vi "UI.vi"(0 "reference in":refnum<class "GUI HIPRESS.lvclass">, 5 "error in (no error)":errorcluster) -> (14 "reference out":refnum<class "GUI HIPRESS.lvclass">, 19 "error out":errorcluster)   [LabVIEW 2019, in "GUI HIPRESS.lvclass"]
uses:
  GUI HIPRESS.lvclass
  GUI_class/GUI.lvclass
  D:/GIT H4000/H4000/src/GUI_class/GUI.lvclass
  d0ca9bf2-7cd9-4c29-a03d-de1c10393a74.vi
  MessageAMC_class/MessageAMC.lvclass
  c2a84178-5316-4673-968e-a9140ec84af1.vi
  7e6ae162-464c-44cf-a5e9-db9ce9dff507.vi
  143f14c2-2a31-4e71-909b-26881bbfe12c.vi
  modbus engine custom/MB_ENGINE_class/Settings.ctl
  modbus engine custom/MB_ENGINE_class/MB_ENGINE.lvclass
  TypeDef/Needle Valve State.ctl
  modbus engine custom/MB_ENGINE_class/Engine State.ctl
  modbus engine custom/MB_ENGINE_class/Engine Alarms.ctl
  TypeDef/Needle Valve Data.ctl
  modbus engine custom/MB_ENGINE_class/Limits Status.ctl
  TypeDef/Step_Name.ctl
  SV_Wrap/SharedVariableWrapper.lvclass
  MessageInterface_class/MessageInterface.lvclass
  b90cc415-26ee-4557-af2e-3b67e66185d6.vi
  TypeDef/AI Statistics Data.ctl
  TypeDef/AI_Data.ctl
  TypeDef/AI_Data_Array.ctl
  D:/GIT H4000/H4000/src/MessageInterface_class/MessageInterface.lvclass
panel:
  in  "Multicolumn Listbox":i32(listbox)=-1
  in  "set":bool
  in  "stop pmg":bool
  in  "start":bool
  in  "step 11":bool
  in  "step 10":bool
  in  "step 8":bool
  in  "step 7":bool
  in  "step 6":bool
  in  "step 5":bool
  in  "step 4":bool
  in  "step 3":bool
  in  "step 2":bool
  in  "step 1":bool
  out "Waveform Chart":T1(graph)
  in  "Setpoint":dbl caption="Уставка [бар]"
  out "Connect":bool
  in  "stop":bool
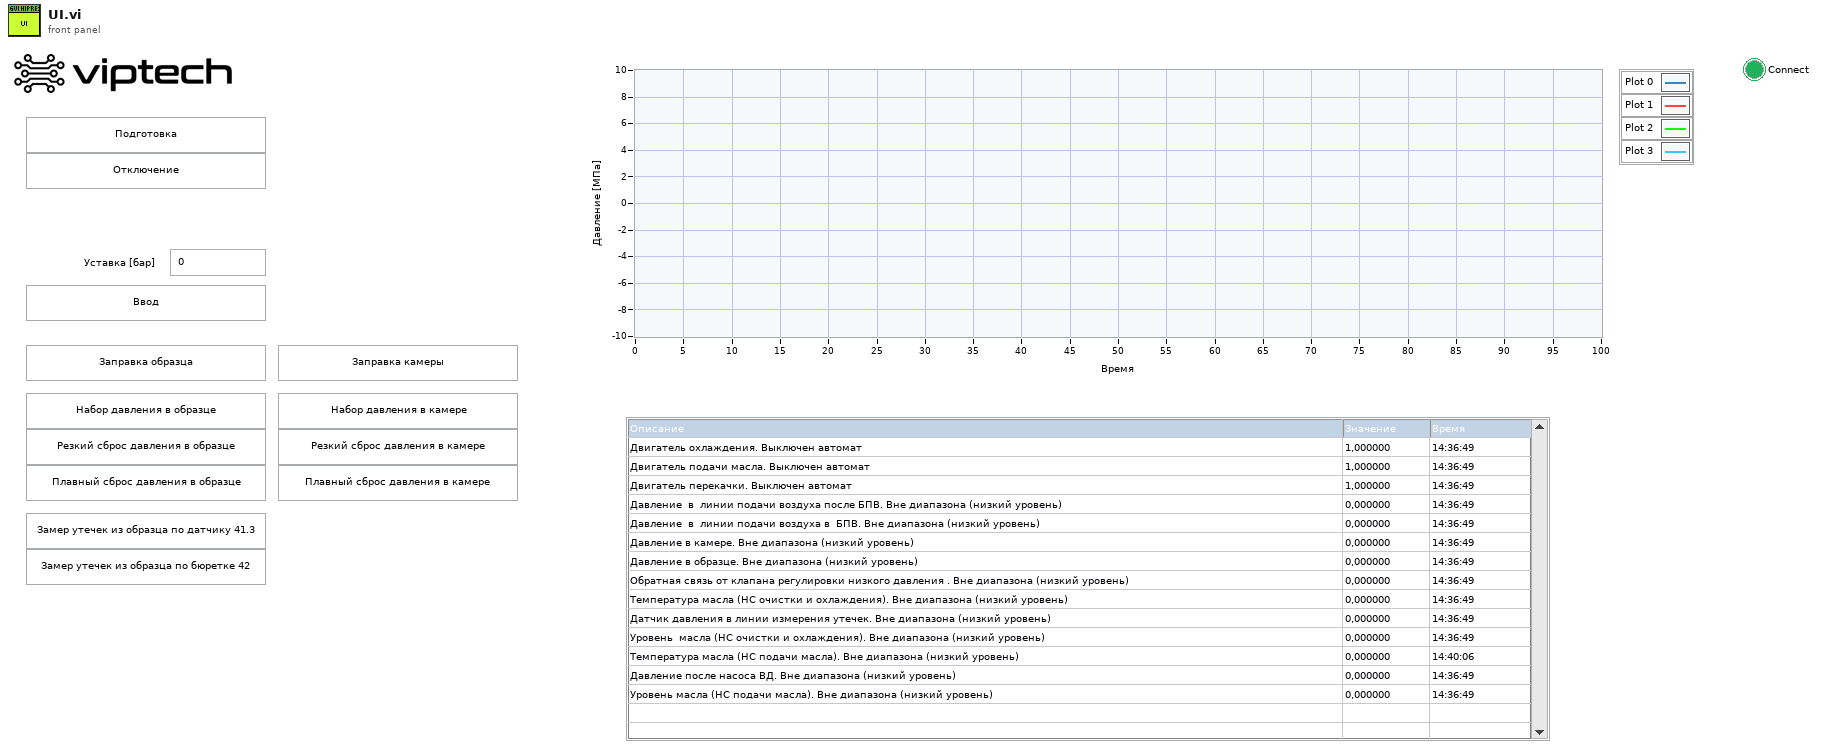
[diagram p1: front panel]
types:
  T1 = cluster{"Setpoint":dbl, "raw mean":dbl, "raw mean":dbl}
  T2 = typedef "Step_Name.ctl" = enum16{"NONE", "Filling DUT", "Filling Chamber", "Pressure Up DUT", "Abrupt Pressure Release DUT", "Smooth Pressure Release DUT", "Pressure Up Chamber", "Abrupt Pressure Release Chamber", "Smooth Pressure Release Chamber", "Measuring leakage sensor 41.3", "Measuring leakage burette 42", "Low Pressure DUT", "Low Pressure Chamber", "Low Pressure HPP", "ALARM", "Open Air", "MicroStep DUT", "MicroStep CMBR", "Stop Pump", "Press Down by Valve DUT"}
  T3 = enum32{"Invalid", "Standard", "Closed", "Hidden", "Minimized", "Maximized"}
  T4 = enum32{"invalid app kind", "Development System", "Run Time System", "Student Edition", "Embedded LabVIEW", "Evaluation", "Custom"}
  T5 = typedef "SharedVariableWrapper.lvclass/Config.ctl" = cluster{"connection str":string, "timeout":dbl, "ip":string}
  T6 = cluster{"Core":cluster{"Current VI Reference":refnum<vi>, "Close Panel on Exit?":bool}, "amc":refnum<class "MessageAMC.lvclass">}
  T7 = cluster{"Current VI Reference":refnum<vi>, "Close Panel on Exit?":bool}
  T8 = typedef "Needle Valve Data.ctl" = cluster{"Engine State":T9, "StateValveModbus":T10, "Alarms":T11, "RAW":i32, "Angele":dbl, "Step":i32, "Encoder":i32, "Kinematic":T12, "Limits":T13, "EncoderMax":i32, "Counter Max Dont Update":i32, "EncoderMin":i32, "Counter Min Dont Update":i32, "Prepere Counter":i32, "STEP INIT":i32, "offset - Angel":dbl}
  T9 = typedef "MB_ENGINE.lvclass/Engine State.ctl" = u16
  T10 = typedef "Needle Valve State.ctl" = enum16{"STOPED", "CLOSED", "OPENED", "OPENING", "CLOSING", "FULL_CLOSE"}
  T11 = typedef "MB_ENGINE.lvclass/Engine Alarms.ctl" = cluster{"OL":bool, "TF":bool, "STL":bool, "OCP":bool, "CPUV":bool, "UVLO":bool, "SPI_ERROR":bool, "Fault":bool, "OL 2":bool, "TF 2":bool, "STL 2":bool, "OCP 2":bool, "CPUV 2":bool, "UVLO 2":bool, "reserved":bool, "InitDone":bool}
  T12 = typedef "MB_ENGINE.lvclass/Settings.ctl" = cluster{"ACC Steps Per Sec^2":u16, "DEC Steps Per Sec^2":u16, "Min Velosity Step Per Sec":u16, "Max Velosity Step Per Sec":u16, "MicroStep":u16}
  T13 = typedef "MB_ENGINE.lvclass/Limits Status.ctl" = cluster{"Fault 2 Switch":bool, "Fault 1 Switch":bool, "Center(Home)":bool, "Lower Limit":bool, "Upper Limit":bool}
  T14 = typedef "AI_Data_Array.ctl" = T15[]
  T15 = typedef "AI_Data.ctl" = cluster{"Stat Data":T16, "OutOfRangeMax":bool, "OutOfRangeMin":bool, "HIHI":bool, "HI":bool, "LO":bool, "LOLO":bool}
  T16 = typedef "AI Statistics Data.ctl" = cluster{"raw mean":dbl, "scl mean":dbl, "raw mean 1Hz":dbl, "scl mean 1Hz":dbl}
  T17 = cluster{"Setpoint":dbl, "scl mean 1Hz":dbl, "scl mean 1Hz":dbl}
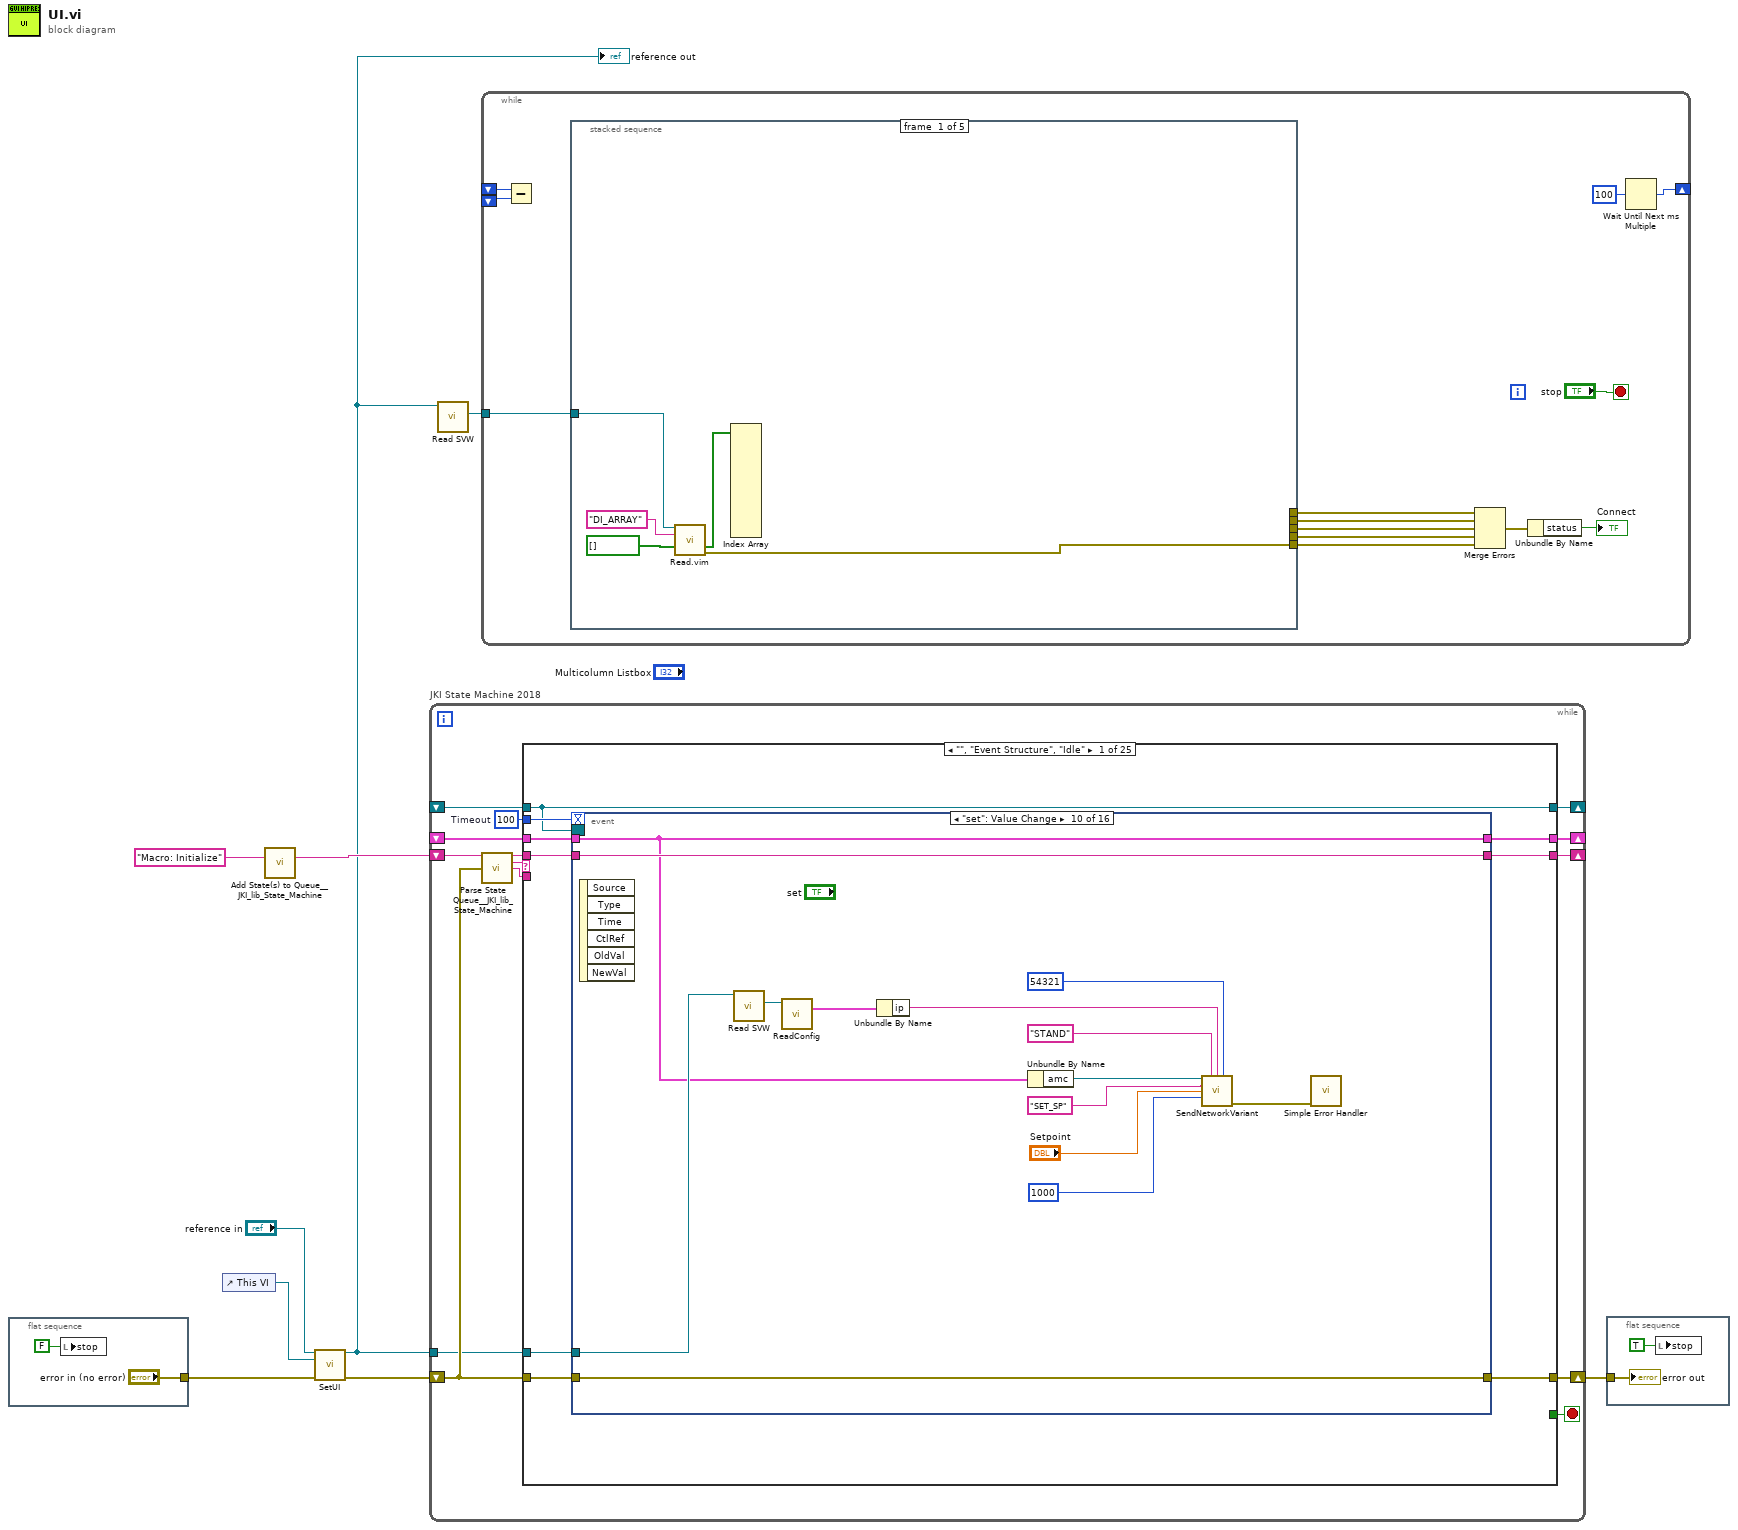
[diagram p0: block diagram]
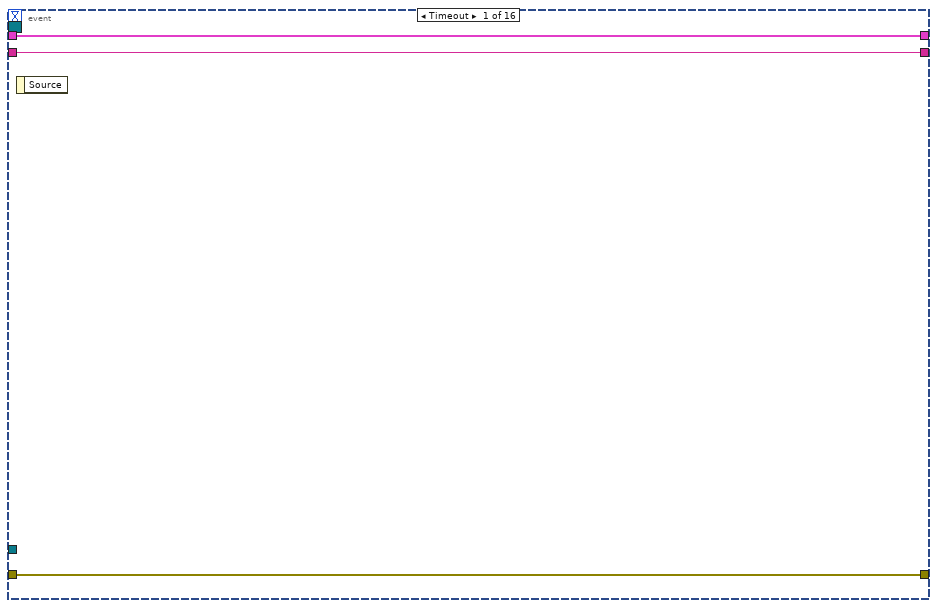
[diagram p2: hidden frame]
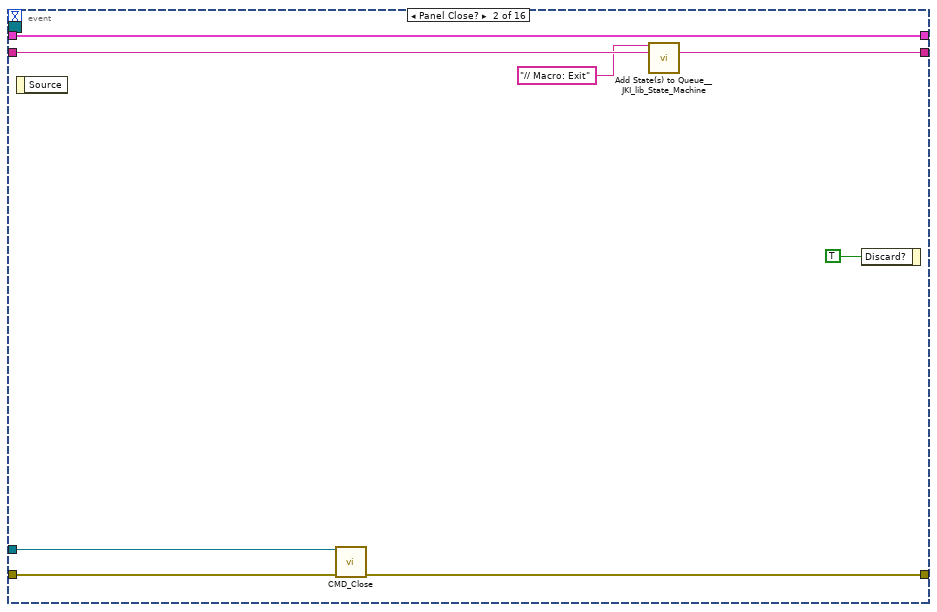
[diagram p3: hidden frame]
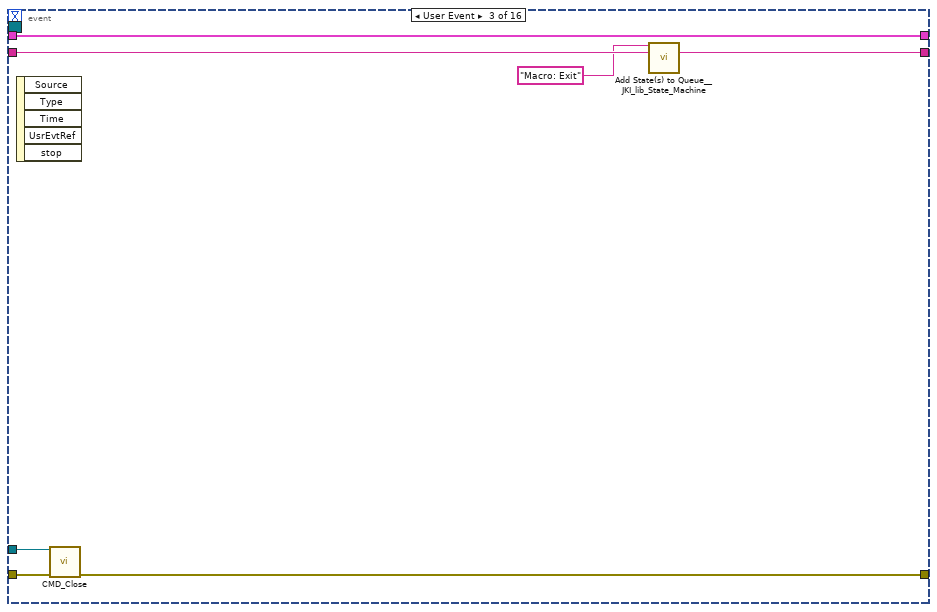
[diagram p4: hidden frame]
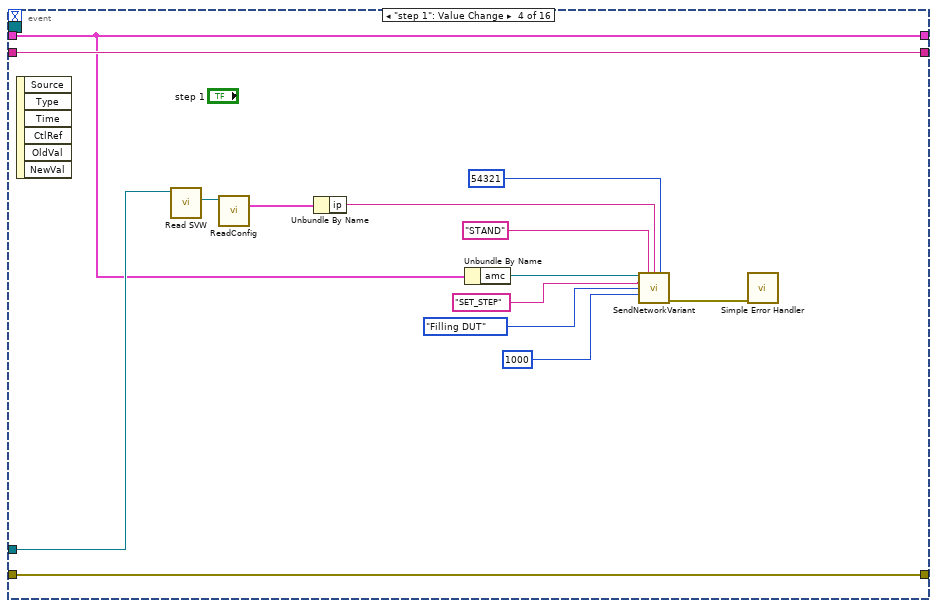
[diagram p5: hidden frame]
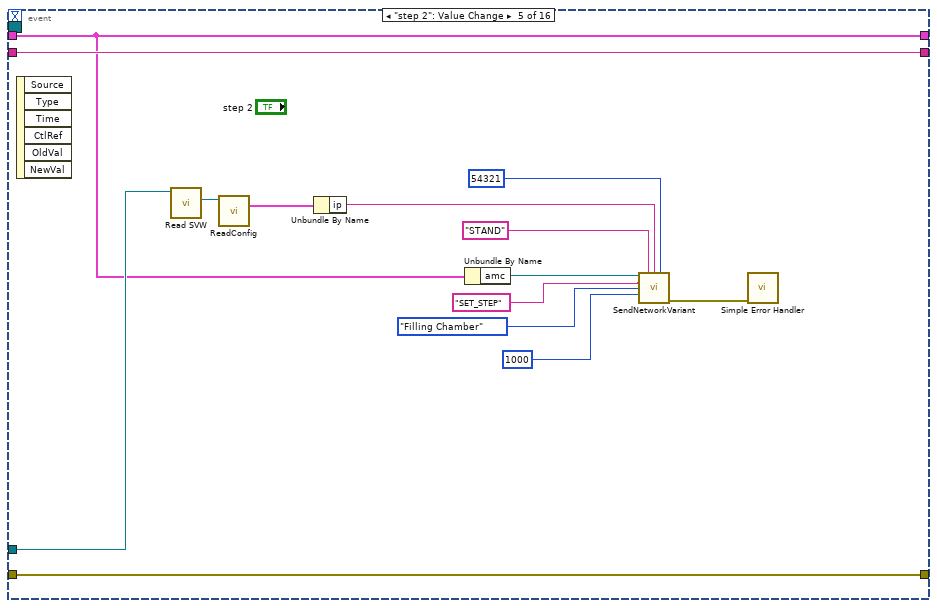
[diagram p6: hidden frame]
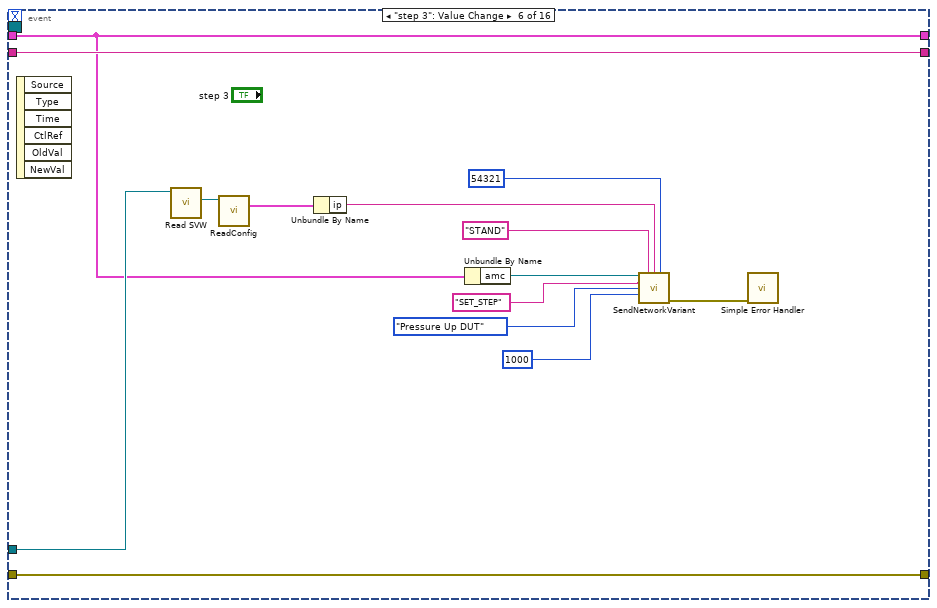
[diagram p7: hidden frame]
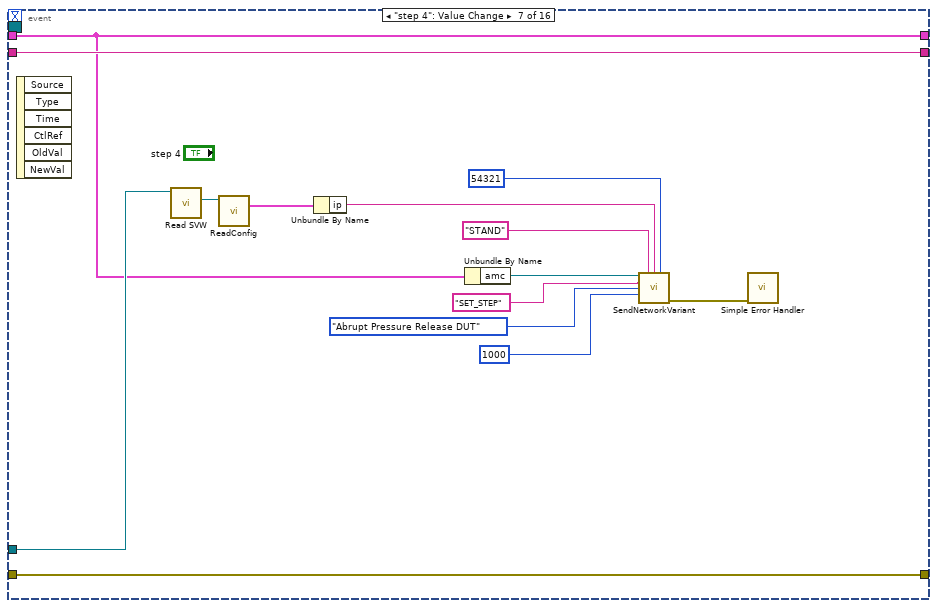
[diagram p8: hidden frame]
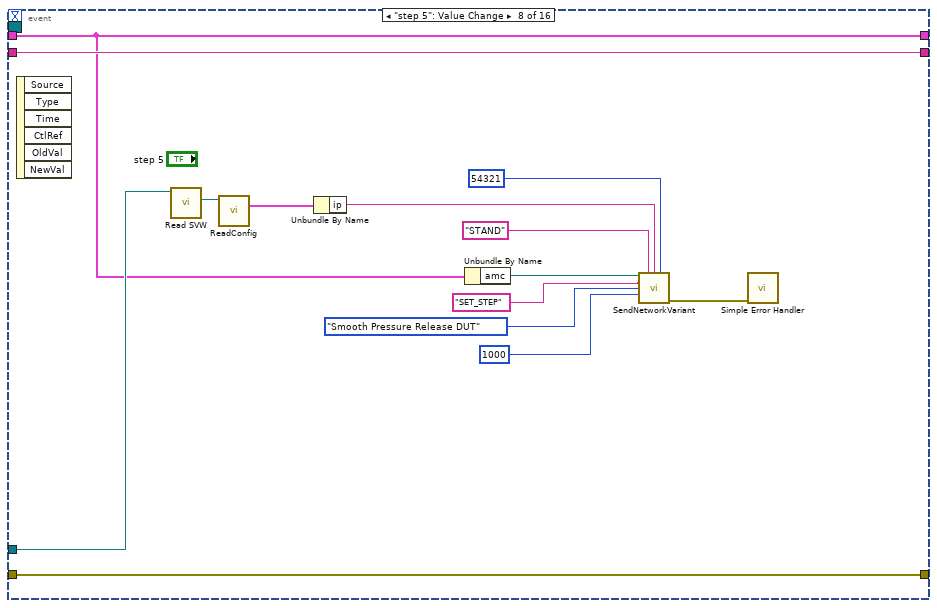
[diagram p9: hidden frame]
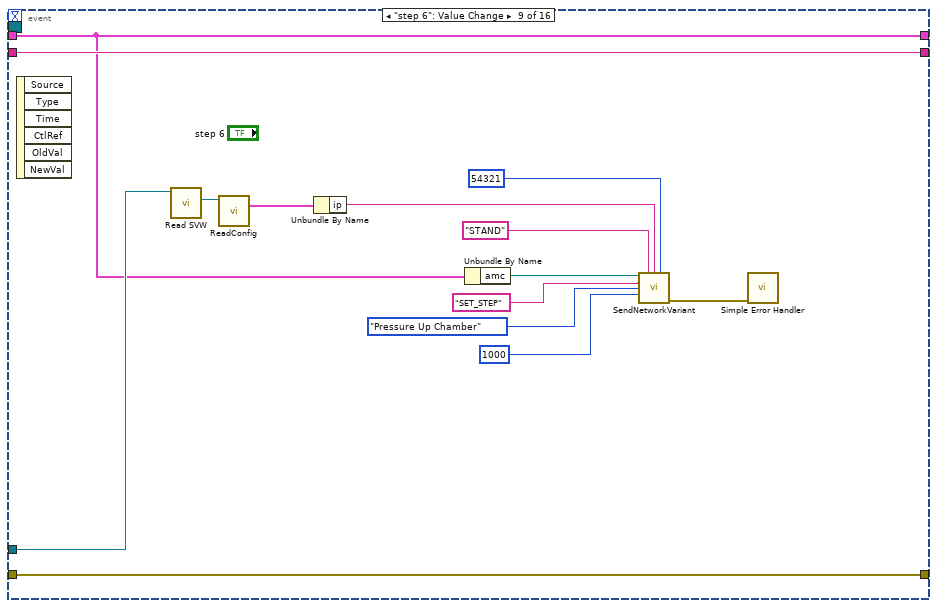
[diagram p10: hidden frame]
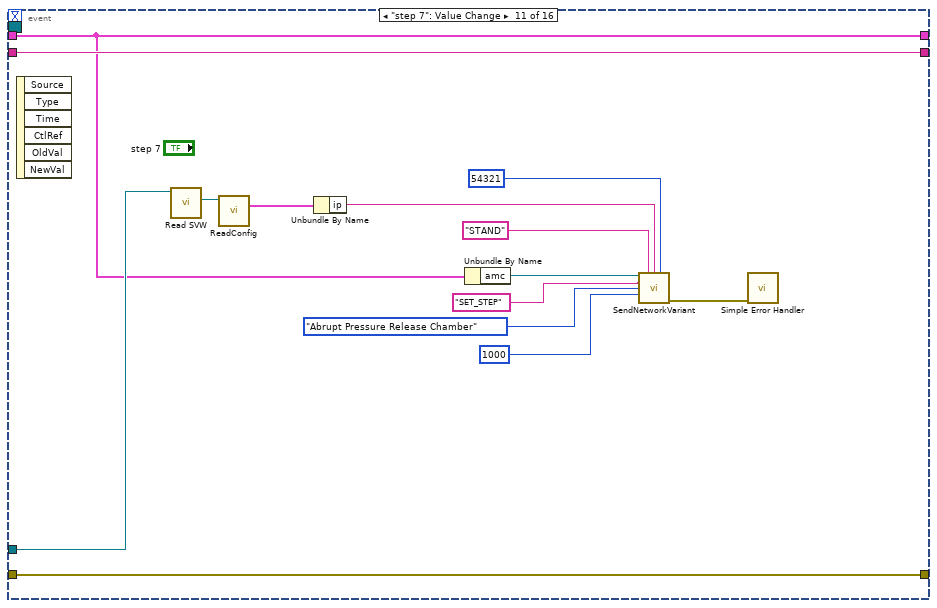
[diagram p11: hidden frame]
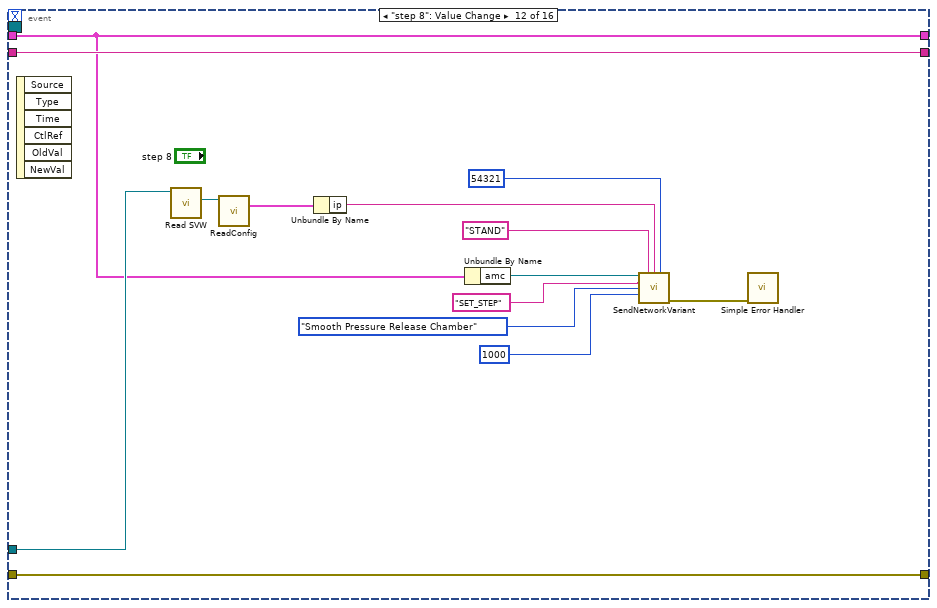
[diagram p12: hidden frame]
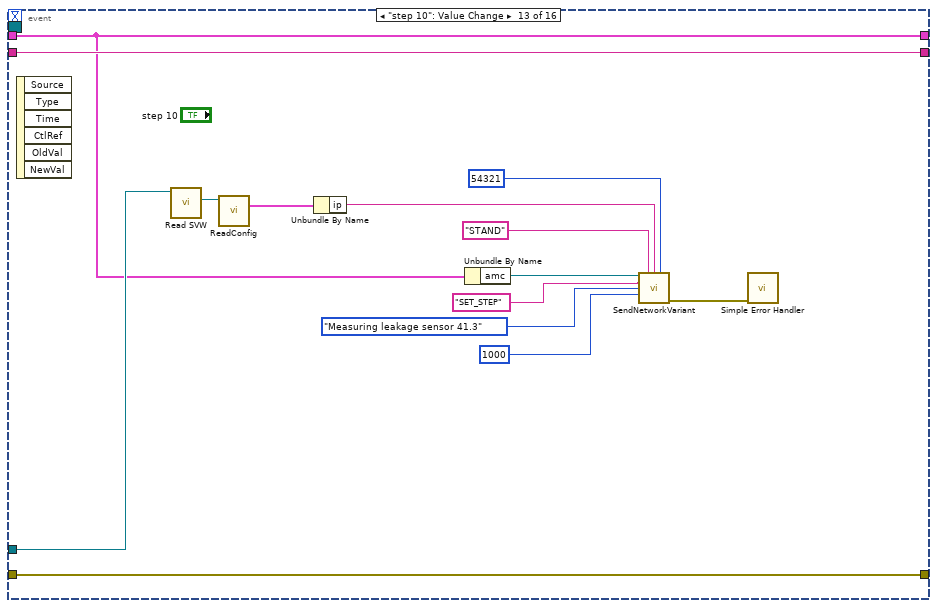
[diagram p13: hidden frame]
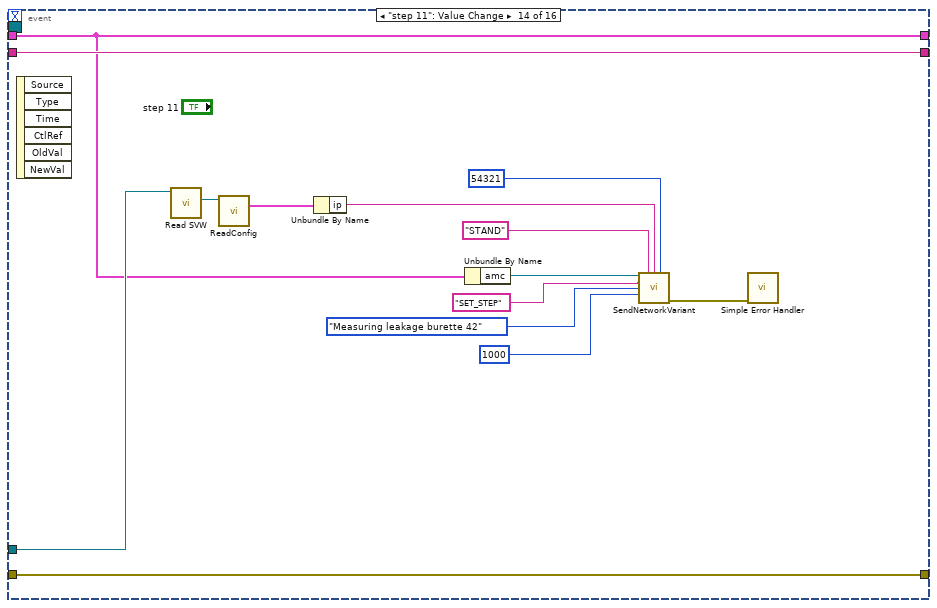
[diagram p14: hidden frame]
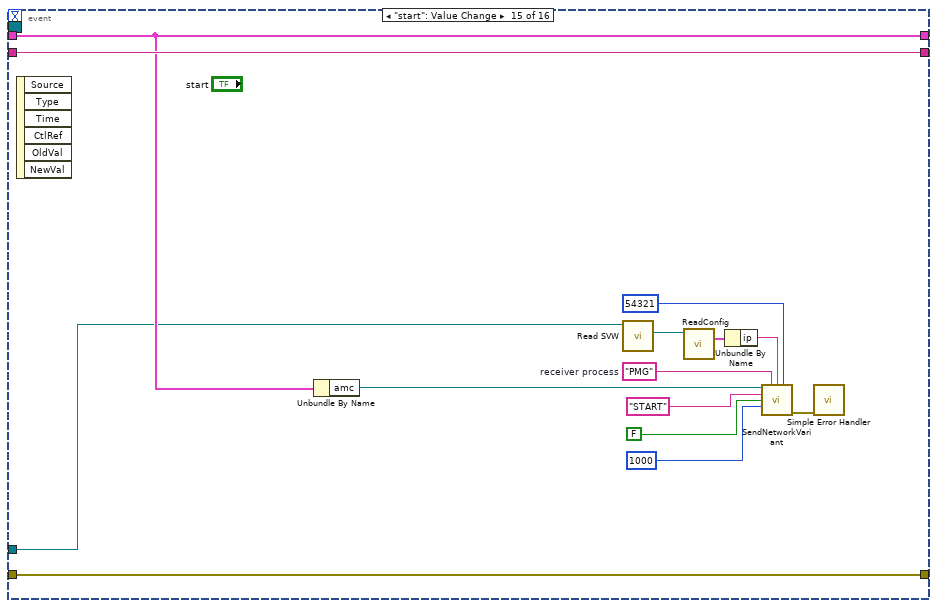
[diagram p15: hidden frame]
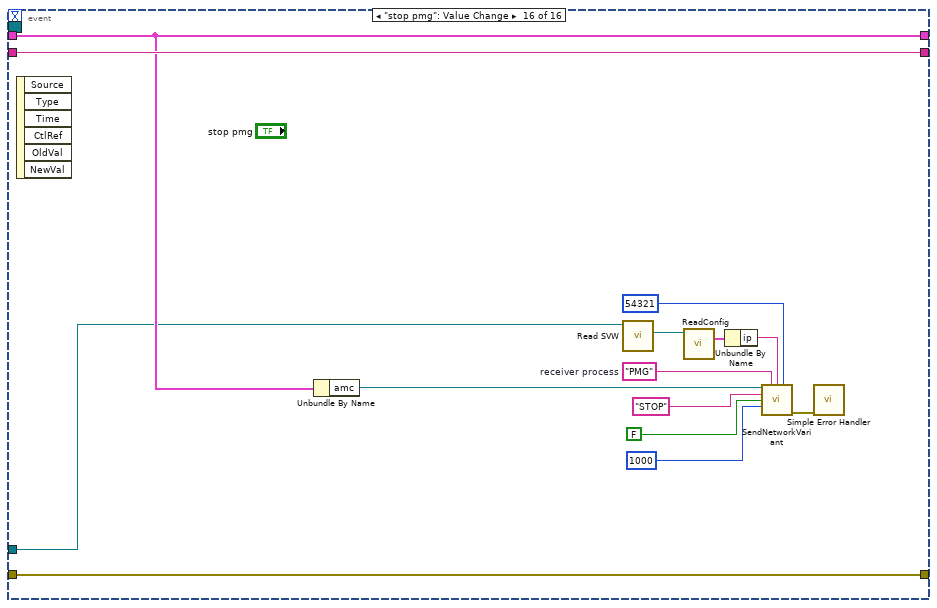
[diagram p16: hidden frame]
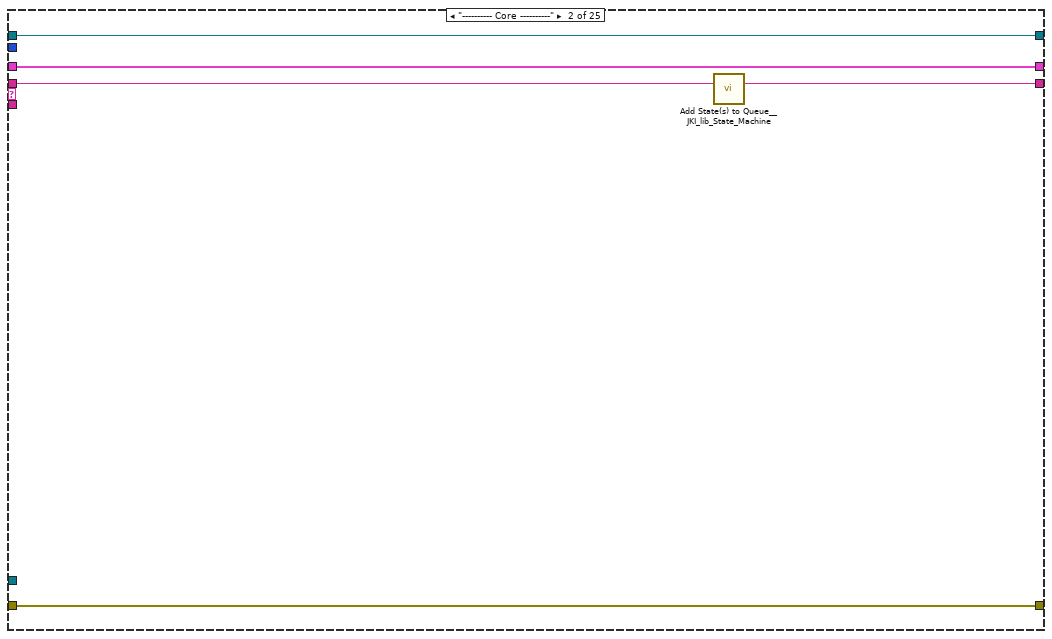
[diagram p17: hidden frame]
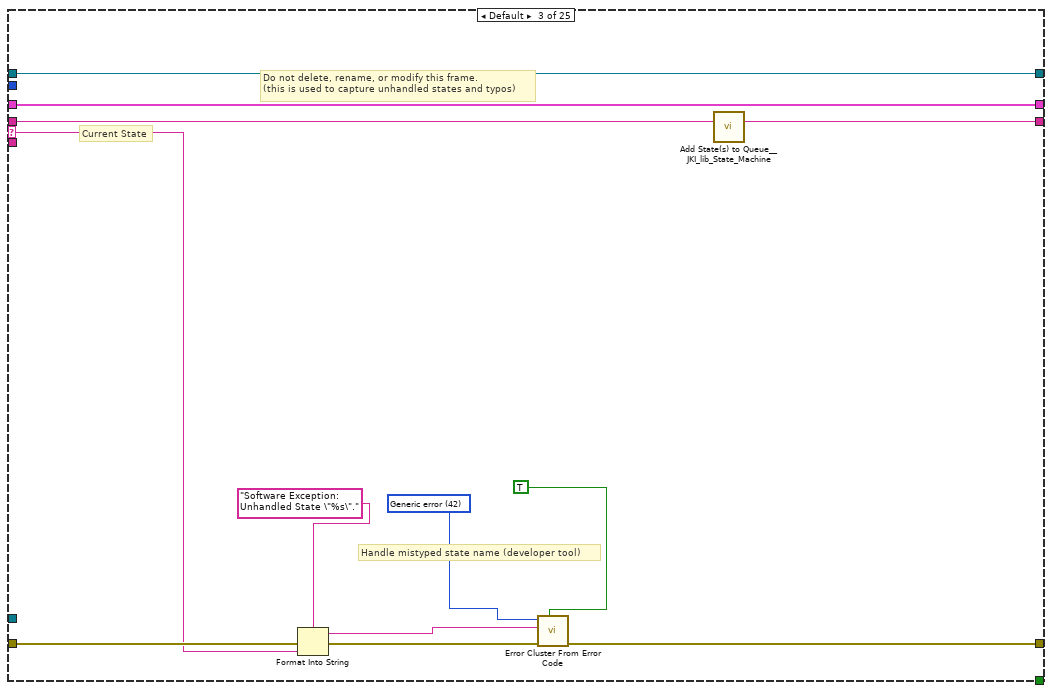
[diagram p18: hidden frame]
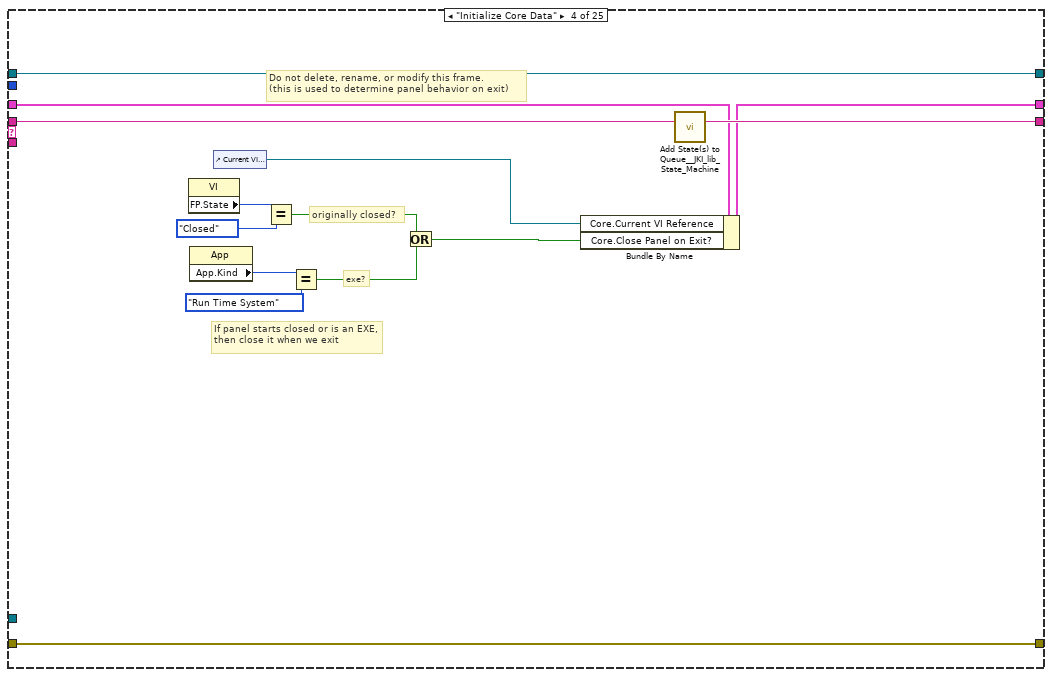
[diagram p19: hidden frame]
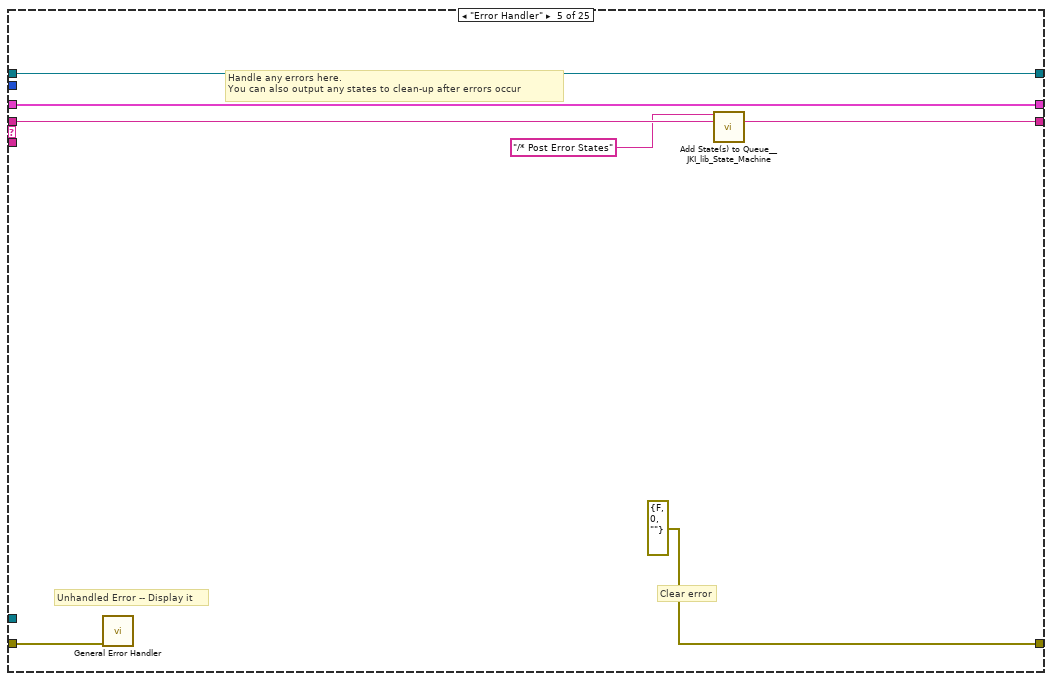
[diagram p20: hidden frame]
diagram:
  n1 = flat-sequence {
    tunnel: ["error in (no error)"] -> w6
    frame #0 {
      n2 = local write "stop"(FALSE ("stop")) -> ()
    }
  }
  n3 = control-ref of="This VI"() -> (w4:refnum<vi>)
  n4 = call <vilib>:"Add State(s) to Queue__JKI_lib_State_Machine.vi"("State(s) in (\"\")"="Macro: Initialize") -> ("States Out"=w9:string)  [unwired: 14 in]
  n5 = call "SetUI.vi"("reference in"="reference in", "UI VI"=w4, "error in (no error)"=w6) -> ("reference out"=w2:refnum<class "GUI HIPRESS.lvclass">, "error out"=w3:errorcluster)  [unwired: 11 in]
  "reference out" <- w2
  n6 = while "JKI State Machine 2018" {
    shift-right: [w18] -> _
    shift-left: _ -> [w17]
    shift-right: [w21] -> w7
    shift-left: w3 -> [w15]
    shift-right: [w20] -> _
    shift-left: w9 -> [w22]
    tunnel: w2 -> [w14]
    shift-right: [w13] -> _
    shift-left: _ -> [w12]
    stop <- w19 stop-if-true
    w16 = 100  # Timeout
    n7 = call <vilib>:"Parse State Queue__JKI_lib_State_Machine.vi"("State Queue"=w22, "Error In (no error)"=w15) -> ("Remaining States"=w24:string, "Current State"=w25:string, "Arguments"=w23:string)  [unwired: 11 in]
    n8 = case shown="\"\", \"Event Structure\", \"Idle\"" w25 {
      selector: w25 -> [_ _ w241 _ _ _ _ _ _ _ _ _ _ _ _ _ _ _ _ _ _ _ _ _ _]
      tunnel: w24 -> [w34 w239 w245 w265 w272 w280 w285 w294 w301 w306 w313 w319 w324 w328 w335 w347 w417 w423 w429 w441 w445 w446 w455 w459 w461]
      tunnel: w23 -> [_ _ _ _ _ _ _ _ _ _ _ _ _ _ w330 w341 _ _ _ _ _ _ _ _ _]
      tunnel: w17 -> [w32 w236 w243 w258 w269 w275 w282 _ w296 w303 w312 w317 w321 w327 w333 w343 w414 w420 w426 w438 w443 w448 w453 w456 w460]
      tunnel: [w31 w237 w247 w262 errorcluster {"status"=FALSE, "code"=0, "source"=""} ("error out") w278 w283 w287 w297 w304 w310 w314 w322 w326 w331 w344 w415 w421 w427 w439 w444 w449 w452 w457 w463] -> w21
      tunnel: w15 -> [w30 w237 w246 w262 w268 w278 w283 w288 w298 w304 w309 w315 w322 w326 w332 w345 w415 w421 w427 w439 w444 w449 w452 w457 w463]
      tunnel: [w33 w238 w244 w264 w271 w279 w284 w294 w300 w305 w313 w318 w323 w328 w334 w346 w416 w422 w428 w440 w445 w447 w455 w459 w461] -> w20
      tunnel: [_ _ _ _ _ TRUE _ _ _ _ _ _ _ _ _ _ _ _ _ _ _ _ _ _ _] -> w19
      tunnel: [w29 w236 w243 w263 w269 w275 w282 w293 w296 w303 w312 w317 w321 w327 w333 w343 w414 w420 w426 w438 w443 w448 w453 w456 w460] -> w18
      tunnel: w16 -> [w28 _ _ _ _ _ _ _ _ _ _ _ _ _ _ _ _ _ _ _ _ _ _ _ _]
      tunnel: w14 -> [w27 _ _ _ _ _ _ _ _ _ w308 _ _ _ _ _ _ _ _ _ _ w450 _ _ _]
      tunnel: [w26 w235 w240 w252 w266 w276 w281 w291 w295 w302 w311 w316 w320 w325 w329 w340 w413 w418 w424 w431 w442 w451 w454 w458 w462] -> w13
      tunnel: w12 -> [w26 w235 w240 w252 w266 w276 w281 w291 w295 w302 _ w316 w320 w325 w329 w340 w413 w418 w424 w431 w442 w451 w454 w458 w462]
      frame "", "Event Structure", "Idle" {
        n9 = event shown="[9] \"set\": Value Change" {
          selector: w26 -> [_ _ _ _ _ _ _ _ _ _ _ _ _ _ _ _]
          dyn-events: _ -> [_ _ _ _ _ _ _ _ _ _ _ _ _ _ _ _]
          timeout: w28 -> [_ _ _ _ _ _ _ _ _ _ _ _ _ _ _ _]
          tunnel: w34 -> [w37 w45 w52 w66 w80 w94 w108 w122 w136 w150 w164 w178 w192 w206 w220 w234]
          tunnel: [w37 w44 w51 w66 w80 w94 w108 w122 w136 w150 w164 w178 w192 w206 w220 w234] -> w33
          tunnel: w32 -> [w35 w43 w50 w60 w74 w88 w102 w116 w130 w144 w158 w172 w186 w200 w208 w222]
          tunnel: [w36 w38 w46 w65 w79 w93 w107 w121 w135 w149 w163 w177 w191 w205 w219 w233] -> w31
          tunnel: w30 -> [w36 w39 w47 w65 w79 w93 w107 w121 w135 w149 w163 w177 w191 w205 w219 w233]
          tunnel: [w35 w43 w50 w60 w74 w88 w102 w116 w130 w144 w158 w172 w186 w200 w208 w222] -> w29
          tunnel: w27 -> [_ w40 w48 w61 w75 w89 w103 w117 w131 w145 w159 w173 w187 w201 w207 w221]
          event Timeout {
            n10 = event-data() -> ()  [unwired: 1 in, 1 out]
          }
          event Panel Close? {
            n11 = event-data() -> ()  [unwired: 1 in, 1 out]
            n12 = call "CMD_Close.vi"("reference in"=w40, "error in (no error)"=w39) -> ("error out"=w38:errorcluster)  [unwired: 12 in, 1 out]
            n13 = call <vilib>:"Add State(s) to Queue__JKI_lib_State_Machine.vi"("State(s) in Front (\"\")"="// Macro: Exit", "State(s) in (\"\")"=w45) -> ("States Out"=w44:string)  [unwired: 13 in]
            n14 = event-data("Discard?"=TRUE) -> ()  [unwired: 1 in, 1 out]
          }
          event User Event {
            n15 = event-data() -> ()  [unwired: 1 in, 5 out]
            n16 = call "CMD_Close.vi"("reference in"=w48, "error in (no error)"=w47) -> ("error out"=w46:errorcluster)  [unwired: 12 in, 1 out]
            n17 = call <vilib>:"Add State(s) to Queue__JKI_lib_State_Machine.vi"("State(s) in Front (\"\")"="Macro: Exit", "State(s) in (\"\")"=w52) -> ("States Out"=w51:string)  [unwired: 13 in]
          }
          event "step 1": Value Change {
            n18 = event-data() -> ()  [unwired: 1 in, 6 out]
            n19 = call "Read SVW.vi"("GUI in"=w61) -> ("SharedVariableWrapper.lvclass"=w64:refnum<class "SharedVariableWrapper.lvclass">)  [unwired: 10 in]
            n20 = call "ReadConfig.vi"("SharedVariableWrapper in"=w64) -> ("config"=w63:T5)  [unwired: 12 in, 2 out]
            n21 = Unbundle By Name(w63) -> ("ip"=w62:string)
            n22 = Unbundle By Name(w60) -> ("amc"=w59:refnum<class "MessageAMC.lvclass">)
            n23 = call "SendNetworkVariant.vi"("reference in"=w59, "receiver process"="STAND", "receiver host"=w62, "receiver port (0)"=u16 54321, "name"="SET_STEP", "data"=Step_Name."Filling DUT" ("stepName"), "timeout (25000 ms)"=1000) -> ("error out"=w56:errorcluster)  [unwired: 6 in, 2 out]
            n24 = call <vilib>:"Simple Error Handler.vi"("error in (no error)"=w56) -> ()  [unwired: 4 in, 5 out]
          }
          event "step 2": Value Change {
            n25 = event-data() -> ()  [unwired: 1 in, 6 out]
            n26 = call "Read SVW.vi"("GUI in"=w75) -> ("SharedVariableWrapper.lvclass"=w78:refnum<class "SharedVariableWrapper.lvclass">)  [unwired: 10 in]
            n27 = call "ReadConfig.vi"("SharedVariableWrapper in"=w78) -> ("config"=w77:T5)  [unwired: 12 in, 2 out]
            n28 = Unbundle By Name(w77) -> ("ip"=w76:string)
            n29 = Unbundle By Name(w74) -> ("amc"=w73:refnum<class "MessageAMC.lvclass">)
            n30 = call "SendNetworkVariant.vi"("reference in"=w73, "receiver process"="STAND", "receiver host"=w76, "receiver port (0)"=u16 54321, "name"="SET_STEP", "data"=Step_Name."Filling Chamber" ("stepName"), "timeout (25000 ms)"=1000) -> ("error out"=w70:errorcluster)  [unwired: 6 in, 2 out]
            n31 = call <vilib>:"Simple Error Handler.vi"("error in (no error)"=w70) -> ()  [unwired: 4 in, 5 out]
          }
          event "step 3": Value Change {
            n32 = event-data() -> ()  [unwired: 1 in, 6 out]
            n33 = call "Read SVW.vi"("GUI in"=w89) -> ("SharedVariableWrapper.lvclass"=w92:refnum<class "SharedVariableWrapper.lvclass">)  [unwired: 10 in]
            n34 = call "ReadConfig.vi"("SharedVariableWrapper in"=w92) -> ("config"=w91:T5)  [unwired: 12 in, 2 out]
            n35 = Unbundle By Name(w91) -> ("ip"=w90:string)
            n36 = Unbundle By Name(w88) -> ("amc"=w87:refnum<class "MessageAMC.lvclass">)
            n37 = call "SendNetworkVariant.vi"("reference in"=w87, "receiver process"="STAND", "receiver host"=w90, "receiver port (0)"=u16 54321, "name"="SET_STEP", "data"=Step_Name."Pressure Up DUT" ("stepName"), "timeout (25000 ms)"=1000) -> ("error out"=w84:errorcluster)  [unwired: 6 in, 2 out]
            n38 = call <vilib>:"Simple Error Handler.vi"("error in (no error)"=w84) -> ()  [unwired: 4 in, 5 out]
          }
          event "step 4": Value Change {
            n39 = event-data() -> ()  [unwired: 1 in, 6 out]
            n40 = call "Read SVW.vi"("GUI in"=w103) -> ("SharedVariableWrapper.lvclass"=w106:refnum<class "SharedVariableWrapper.lvclass">)  [unwired: 10 in]
            n41 = call "ReadConfig.vi"("SharedVariableWrapper in"=w106) -> ("config"=w105:T5)  [unwired: 12 in, 2 out]
            n42 = Unbundle By Name(w105) -> ("ip"=w104:string)
            n43 = Unbundle By Name(w102) -> ("amc"=w101:refnum<class "MessageAMC.lvclass">)
            n44 = call "SendNetworkVariant.vi"("reference in"=w101, "receiver process"="STAND", "receiver host"=w104, "receiver port (0)"=u16 54321, "name"="SET_STEP", "data"=Step_Name."Abrupt Pressure Release DUT" ("stepName"), "timeout (25000 ms)"=1000) -> ("error out"=w98:errorcluster)  [unwired: 6 in, 2 out]
            n45 = call <vilib>:"Simple Error Handler.vi"("error in (no error)"=w98) -> ()  [unwired: 4 in, 5 out]
          }
          event "step 5": Value Change {
            n46 = event-data() -> ()  [unwired: 1 in, 6 out]
            n47 = call "Read SVW.vi"("GUI in"=w117) -> ("SharedVariableWrapper.lvclass"=w120:refnum<class "SharedVariableWrapper.lvclass">)  [unwired: 10 in]
            n48 = call "ReadConfig.vi"("SharedVariableWrapper in"=w120) -> ("config"=w119:T5)  [unwired: 12 in, 2 out]
            n49 = Unbundle By Name(w119) -> ("ip"=w118:string)
            n50 = Unbundle By Name(w116) -> ("amc"=w115:refnum<class "MessageAMC.lvclass">)
            n51 = call "SendNetworkVariant.vi"("reference in"=w115, "receiver process"="STAND", "receiver host"=w118, "receiver port (0)"=u16 54321, "name"="SET_STEP", "data"=Step_Name."Smooth Pressure Release DUT" ("stepName"), "timeout (25000 ms)"=1000) -> ("error out"=w112:errorcluster)  [unwired: 6 in, 2 out]
            n52 = call <vilib>:"Simple Error Handler.vi"("error in (no error)"=w112) -> ()  [unwired: 4 in, 5 out]
          }
          event "step 6": Value Change {
            n53 = event-data() -> ()  [unwired: 1 in, 6 out]
            n54 = call "Read SVW.vi"("GUI in"=w131) -> ("SharedVariableWrapper.lvclass"=w134:refnum<class "SharedVariableWrapper.lvclass">)  [unwired: 10 in]
            n55 = call "ReadConfig.vi"("SharedVariableWrapper in"=w134) -> ("config"=w133:T5)  [unwired: 12 in, 2 out]
            n56 = Unbundle By Name(w133) -> ("ip"=w132:string)
            n57 = Unbundle By Name(w130) -> ("amc"=w129:refnum<class "MessageAMC.lvclass">)
            n58 = call "SendNetworkVariant.vi"("reference in"=w129, "receiver process"="STAND", "receiver host"=w132, "receiver port (0)"=u16 54321, "name"="SET_STEP", "data"=Step_Name."Pressure Up Chamber" ("stepName"), "timeout (25000 ms)"=1000) -> ("error out"=w126:errorcluster)  [unwired: 6 in, 2 out]
            n59 = call <vilib>:"Simple Error Handler.vi"("error in (no error)"=w126) -> ()  [unwired: 4 in, 5 out]
          }
          event "set": Value Change {
            n60 = event-data() -> ()  [unwired: 1 in, 6 out]
            n61 = call "Read SVW.vi"("GUI in"=w145) -> ("SharedVariableWrapper.lvclass"=w148:refnum<class "SharedVariableWrapper.lvclass">)  [unwired: 10 in]
            n62 = call "ReadConfig.vi"("SharedVariableWrapper in"=w148) -> ("config"=w147:T5)  [unwired: 12 in, 2 out]
            n63 = Unbundle By Name(w147) -> ("ip"=w146:string)
            n64 = Unbundle By Name(w144) -> ("amc"=w143:refnum<class "MessageAMC.lvclass">)
            n65 = call "SendNetworkVariant.vi"("reference in"=w143, "receiver process"="STAND", "receiver host"=w146, "receiver port (0)"=u16 54321, "name"="SET_SP", "data"="Setpoint", "timeout (25000 ms)"=1000) -> ("error out"=w140:errorcluster)  [unwired: 6 in, 2 out]
            n66 = call <vilib>:"Simple Error Handler.vi"("error in (no error)"=w140) -> ()  [unwired: 4 in, 5 out]
          }
          event "step 7": Value Change {
            n67 = event-data() -> ()  [unwired: 1 in, 6 out]
            n68 = call "Read SVW.vi"("GUI in"=w159) -> ("SharedVariableWrapper.lvclass"=w162:refnum<class "SharedVariableWrapper.lvclass">)  [unwired: 10 in]
            n69 = call "ReadConfig.vi"("SharedVariableWrapper in"=w162) -> ("config"=w161:T5)  [unwired: 12 in, 2 out]
            n70 = Unbundle By Name(w161) -> ("ip"=w160:string)
            n71 = Unbundle By Name(w158) -> ("amc"=w157:refnum<class "MessageAMC.lvclass">)
            n72 = call "SendNetworkVariant.vi"("reference in"=w157, "receiver process"="STAND", "receiver host"=w160, "receiver port (0)"=u16 54321, "name"="SET_STEP", "data"=Step_Name."Abrupt Pressure Release Chamber" ("stepName"), "timeout (25000 ms)"=1000) -> ("error out"=w154:errorcluster)  [unwired: 6 in, 2 out]
            n73 = call <vilib>:"Simple Error Handler.vi"("error in (no error)"=w154) -> ()  [unwired: 4 in, 5 out]
          }
          event "step 8": Value Change {
            n74 = event-data() -> ()  [unwired: 1 in, 6 out]
            n75 = call "Read SVW.vi"("GUI in"=w173) -> ("SharedVariableWrapper.lvclass"=w176:refnum<class "SharedVariableWrapper.lvclass">)  [unwired: 10 in]
            n76 = call "ReadConfig.vi"("SharedVariableWrapper in"=w176) -> ("config"=w175:T5)  [unwired: 12 in, 2 out]
            n77 = Unbundle By Name(w175) -> ("ip"=w174:string)
            n78 = Unbundle By Name(w172) -> ("amc"=w171:refnum<class "MessageAMC.lvclass">)
            n79 = call "SendNetworkVariant.vi"("reference in"=w171, "receiver process"="STAND", "receiver host"=w174, "receiver port (0)"=u16 54321, "name"="SET_STEP", "data"=Step_Name."Smooth Pressure Release Chamber" ("stepName"), "timeout (25000 ms)"=1000) -> ("error out"=w168:errorcluster)  [unwired: 6 in, 2 out]
            n80 = call <vilib>:"Simple Error Handler.vi"("error in (no error)"=w168) -> ()  [unwired: 4 in, 5 out]
          }
          event "step 10": Value Change {
            n81 = event-data() -> ()  [unwired: 1 in, 6 out]
            n82 = call "Read SVW.vi"("GUI in"=w187) -> ("SharedVariableWrapper.lvclass"=w190:refnum<class "SharedVariableWrapper.lvclass">)  [unwired: 10 in]
            n83 = call "ReadConfig.vi"("SharedVariableWrapper in"=w190) -> ("config"=w189:T5)  [unwired: 12 in, 2 out]
            n84 = Unbundle By Name(w189) -> ("ip"=w188:string)
            n85 = Unbundle By Name(w186) -> ("amc"=w185:refnum<class "MessageAMC.lvclass">)
            n86 = call "SendNetworkVariant.vi"("reference in"=w185, "receiver process"="STAND", "receiver host"=w188, "receiver port (0)"=u16 54321, "name"="SET_STEP", "data"=Step_Name."Measuring leakage sensor 41.3" ("stepName"), "timeout (25000 ms)"=1000) -> ("error out"=w182:errorcluster)  [unwired: 6 in, 2 out]
            n87 = call <vilib>:"Simple Error Handler.vi"("error in (no error)"=w182) -> ()  [unwired: 4 in, 5 out]
          }
          event "step 11": Value Change {
            n88 = event-data() -> ()  [unwired: 1 in, 6 out]
            n89 = call "Read SVW.vi"("GUI in"=w201) -> ("SharedVariableWrapper.lvclass"=w204:refnum<class "SharedVariableWrapper.lvclass">)  [unwired: 10 in]
            n90 = call "ReadConfig.vi"("SharedVariableWrapper in"=w204) -> ("config"=w203:T5)  [unwired: 12 in, 2 out]
            n91 = Unbundle By Name(w203) -> ("ip"=w202:string)
            n92 = Unbundle By Name(w200) -> ("amc"=w199:refnum<class "MessageAMC.lvclass">)
            n93 = call "SendNetworkVariant.vi"("reference in"=w199, "receiver process"="STAND", "receiver host"=w202, "receiver port (0)"=u16 54321, "name"="SET_STEP", "data"=Step_Name."Measuring leakage burette 42" ("stepName"), "timeout (25000 ms)"=1000) -> ("error out"=w196:errorcluster)  [unwired: 6 in, 2 out]
            n94 = call <vilib>:"Simple Error Handler.vi"("error in (no error)"=w196) -> ()  [unwired: 4 in, 5 out]
          }
          event "start": Value Change {
            w209 = "PMG"  # receiver process
            n95 = event-data() -> ()  [unwired: 1 in, 6 out]
            n96 = Unbundle By Name(w208) -> ("amc"=w213:refnum<class "MessageAMC.lvclass">)
            n97 = call "Read SVW.vi"("GUI in"=w207) -> ("SharedVariableWrapper.lvclass"=w215:refnum<class "SharedVariableWrapper.lvclass">)  [unwired: 10 in]
            n98 = call "ReadConfig.vi"("SharedVariableWrapper in"=w215) -> ("config"=w214:T5)  [unwired: 12 in, 2 out]
            n99 = Unbundle By Name(w214) -> ("ip"=w212:string)
            n100 = call "SendNetworkVariant.vi"("reference in"=w213, "receiver process"=w209, "receiver host"=w212, "receiver port (0)"=u16 54321, "name"="START", "data"=FALSE, "timeout (25000 ms)"=1000) -> ("error out"=w210:errorcluster)  [unwired: 6 in, 2 out]
            n101 = call <vilib>:"Simple Error Handler.vi"("error in (no error)"=w210) -> ()  [unwired: 4 in, 5 out]
          }
          event "stop pmg": Value Change {
            w223 = "PMG"  # receiver process
            n102 = event-data() -> ()  [unwired: 1 in, 6 out]
            n103 = Unbundle By Name(w222) -> ("amc"=w227:refnum<class "MessageAMC.lvclass">)
            n104 = call "Read SVW.vi"("GUI in"=w221) -> ("SharedVariableWrapper.lvclass"=w229:refnum<class "SharedVariableWrapper.lvclass">)  [unwired: 10 in]
            n105 = call "ReadConfig.vi"("SharedVariableWrapper in"=w229) -> ("config"=w228:T5)  [unwired: 12 in, 2 out]
            n106 = Unbundle By Name(w228) -> ("ip"=w226:string)
            n107 = call "SendNetworkVariant.vi"("reference in"=w227, "receiver process"=w223, "receiver host"=w226, "receiver port (0)"=u16 54321, "name"="STOP", "data"=FALSE, "timeout (25000 ms)"=1000) -> ("error out"=w224:errorcluster)  [unwired: 6 in, 2 out]
            n108 = call <vilib>:"Simple Error Handler.vi"("error in (no error)"=w224) -> ()  [unwired: 4 in, 5 out]
          }
        }
      }
      frame "---------- Core ----------" {
        n109 = call <vilib>:"Add State(s) to Queue__JKI_lib_State_Machine.vi"("State(s) in (\"\")"=w239) -> ("States Out"=w238:string)  [unwired: 14 in]
      }
      frame Default {
        w250 = 42 items=["No error", "Argument error", "Memory is full", "Out of zone", "End of file", "File already open", "Generic file I/O error", "File not found", "File permission error", "Disk is full", "Duplicate path", "Too many files open", "System feature not enabled", "Resource file not found", "Cannot add resource", "Resource not found", "Image not found", "Image memory error", "Pen does not exist", "Config type invalid", "Config token not found", "Config parse error", "Config memory error", "Bad external code format", "Bad external code offset", "External code not present", "Null window", "Destroy window error", "Null menu", "Print aborted", "Bad print record", "Print driver error", "Windows error during printing", "Memory error during printing", "Print dialog error", "Generic print error", "Invalid device refnum", "Device not found", "Device parameter error", "Device unit error", "Cannot open device", "Device call aborted", "Generic error", "Cancelled by user", "Object ID too low", "Object ID too high", "Object not in heap", "Unknown heap", "Unknown object (invalid DefProc)", "Unknown object (DefProc not in table)", "Message out of range", "Invalid (null) method", "Unknown message", "Manager call not supported", "Bad address", "Network operation in progress", "Network operation timed out", "Connection is busy", "Network attribute not supported", "Network error", "Address in use", "System out of memory", "Connection aborted", "Connection refused", "Not connected", "Already connected", "Connection closed", "Initialization error (interapplication manager)", "Bad occurrence", "Wait on unbound occurrence handler", "Occurrence queue overflow", "Datalog type conflict", "Unused", "Unrecognized type (interapplication manager)", "Memory corrupt", "Failed to make temporary DLL", "Old CIN version", "Drag socket not found", "Failed to load drop-object", "Failed to register OLE object", "Failed to release OLE object", "Format specifier type mismatch", "Unknown format specifier", "Too few format specifiers", "Too many format specifiers", "Scan failed", "Newer CIN version", "Error converting to variant", "Runtime menu error", "Password tampered", "Variant attribute not found", "Incompatible variant data type", "Event data is not available", "Event Store is not present", "Occurrence is not found", "Event Queue is not created", "Event info is not available", "Refnum passed is NULL", "Error retrieving Class GUID", "Error retrieving CoClass GUID", "Error retrieving TypeLib GUID.", "Bad built application magic bytes.", "Specific driver is different from the specific driver associated with the Logical Name.", "There is no session opened to the class driver.", "Max Error", "MAX - Error with config objects", "MAX - Error loading configuration", "MAX - Group not supported"]
        # "Current State"
        # "Do not delete, rename, or modify this frame.\n(this is used to capture unhandled states and typos)"
        # "Handle mistyped state name (developer tool)"
        n110 = Format Into String(format string="Software Exception: Unhandled State \"%s\"." ("message"), error in=w246, w241) -> (resulting string=w249:string, error out=w248:errorcluster)  [unwired: 1 in]
        n111 = call <vilib>:"Error Cluster From Error Code.vi"("show call chain? (False)"=TRUE, "error in (no error)"=w248, "error message (\"\")"=w249, "error code (0)"=w250) -> ("error out"=w247:errorcluster)  [unwired: 5 in]
        n112 = call <vilib>:"Add State(s) to Queue__JKI_lib_State_Machine.vi"("State(s) in (\"\")"=w245) -> ("States Out"=w244:string)  [unwired: 14 in]
      }
      frame "Initialize Core Data" {
        # "Do not delete, rename, or modify this frame.\n(this is used to determine panel behavior on exit)"
        # "originally closed?"
        # "exe?"
        # "If panel starts closed or is an EXE, then close it when we exit"
        n113 = property class="VI"() -> ("FP.State"=w255:T3)  [unwired: 2 in, 2 out]
        n114 = property class="App"() -> ("App.Kind"=w261:T4)  [unwired: 2 in, 2 out]
        n115 = control-ref of="Current VI Reference"() -> (w256:refnum<vi>)
        n116 = Equal?(x=w255, y=T3."Closed" ("Front Panel Window:State")) -> (x = y?=w253:bool)
        n117 = Equal?(x=w261, y=T4."Run Time System" ("Application:Kind")) -> (x = y?=w259:bool)
        n118 = Or(x=w253, y=w259) -> (x .or. y?=w257:bool)
        n119 = Bundle By Name(cluster=w258, "Core.Current VI Reference"=w256, "Core.Close Panel on Exit?"=w257) -> (w263:T6)
        n120 = call <vilib>:"Add State(s) to Queue__JKI_lib_State_Machine.vi"("State(s) in (\"\")"=w265) -> ("States Out"=w264:string)  [unwired: 14 in]
      }
      frame "Error Handler" {
        # "Unhandled Error -- Display it"
        # "Handle any errors here.\nYou can also output any states to clean-up after errors occur"
        # "Clear error"
        n121 = call <vilib>:"General Error Handler.vi"("error in (no error)"=w268) -> ()  [unwired: 10 in, 5 out]
        n122 = call <vilib>:"Add State(s) to Queue__JKI_lib_State_Machine.vi"("State(s) in Front (\"\")"="/* Post Error States", "State(s) in (\"\")"=w272) -> ("States Out"=w271:string)  [unwired: 13 in]
      }
      frame "Exit" {
        n123 = Unbundle By Name(w275) -> ("amc"=w274:refnum<class "MessageAMC.lvclass">)
        n124 = call-dynamic "Destroy.vi"("reference in"=w274) -> ("error out"=w273:errorcluster)  [unwired: 17 in, 1 out]
        n125 = call <vilib>:"Clear Errors.vi"("error in (no error)"=w273) -> ()  [unwired: 5 in, 2 out]
        n126 = call <vilib>:"Add State(s) to Queue__JKI_lib_State_Machine.vi"("State(s) in (\"\")"=w280) -> ("States Out"=w279:string)  [unwired: 14 in]
      }
      frame "---------- Data ----------" {
        # "Do not put any code in this frame.\n(It is a separator no-op. You can make a copy of this frame to create a new Data frame)"
        n127 = call <vilib>:"Add State(s) to Queue__JKI_lib_State_Machine.vi"("State(s) in (\"\")"=w285) -> ("States Out"=w284:string)  [unwired: 14 in]
      }
      frame "Data: Initialize" {
        w292 = T7 {"Current VI Reference"=refnum, "Close Panel on Exit?"=FALSE}  # Core
        n128 = call "MessageAMC_Create.vi"("reference in"=refnum<class "MessageAMC.lvclass"> refnum, "error in (no error)"=w288, "message queue name"="GUI_TEST_CHNLS") -> ("amc"=w289:refnum<class "MessageAMC.lvclass">, "error out"=w287:errorcluster)  [unwired: 15 in]
        n129 = Bundle("Core"=w292, "amc"=w289) -> (w293:T6)  [unwired: 1 in]
      }
      frame "Data: Cleanup" {
        # "Cleanup any data and references, here.\n(this is called automatically, by the Macro: Exit)"
        n130 = Unbundle By Name(w296) -> ("Core.Current VI Reference"=w299:refnum<vi>)
        n131 = Close Reference(reference=w299, error in (no error)=w298) -> (error out=w297:errorcluster)
        n132 = call <vilib>:"Add State(s) to Queue__JKI_lib_State_Machine.vi"("State(s) in (\"\")"=w301) -> ("States Out"=w300:string)  [unwired: 14 in]
      }
      frame "---------- Events ----------" {
        # "Do not put any code in this frame.\n(It is a separator no-op. You can make a copy of this frame to create a new UI frame)"
        n133 = call <vilib>:"Add State(s) to Queue__JKI_lib_State_Machine.vi"("State(s) in (\"\")"=w306) -> ("States Out"=w305:string)  [unwired: 14 in]
      }
      frame "Events: Register" {
        n134 = call "Read stop event.vi"("GUI in"=w308) -> ("stop event"=w307:refnum<user-event>)  [unwired: 8 in, 2 out]
        n135 = register-events(error in=w309, w307) -> (reference out=w311:refnum<event-registration>, error out=w310:errorcluster)  [unwired: 1 in]
      }
      frame "Events: Unregister" {
        # "Do not put any code in this frame.\n(It is a separator no-op. You can make a copy of this frame to create a new UI frame)"
        n136 = Unregister For Events(event registration refnum=w316, error in=w315) -> (error out=w314:errorcluster)
        n137 = call <vilib>:"Add State(s) to Queue__JKI_lib_State_Machine.vi"("State(s) in (\"\")"=w319) -> ("States Out"=w318:string)  [unwired: 14 in]
      }
      frame "---------- UI ----------" {
        # "Do not put any code in this frame.\n(It is a separator no-op. You can make a copy of this frame to create a new UI frame)"
        n138 = call <vilib>:"Add State(s) to Queue__JKI_lib_State_Machine.vi"("State(s) in (\"\")"=w324) -> ("States Out"=w323:string)  [unwired: 14 in]
      }
      frame "UI: Initialize" {
      }
      frame "UI: Cursor Set" {
        # "Argument"
        # "Set and Unset Cursor Busy.\n(Usage: \"UI: Cursor Set >> Busy|Idle\")"
        n139 = case shown="\"Idle\", Default" w330 {
          tunnel: w332 -> [w337 w339]
          tunnel: [w336 w338] -> w331
          frame "Idle", Default {
            n140 = call <vilib>:"Unset Busy.vi"("error in (no error)"=w337) -> ("error out"=w336:errorcluster)  [unwired: 10 in]
          }
          frame "Busy" {
            n141 = call <vilib>:"Set Busy.vi"("error in (no error)"=w339) -> ("error out"=w338:errorcluster)  [unwired: 9 in, 1 out]
          }
        }
        n142 = call <vilib>:"Add State(s) to Queue__JKI_lib_State_Machine.vi"("State(s) in (\"\")"=w335) -> ("States Out"=w334:string)  [unwired: 14 in]
      }
      frame "UI: Front Panel State" {
        # "Argument"
        # "Set Front Panel Open or Closed\n(Usage: \"UI: Front Panel State >> Open|Close\")"
        n143 = Unbundle By Name(w343) -> ("Core.Current VI Reference"=w342:refnum<vi>)
        n144 = case shown="\"Minimize\", \"Minimized\"" w341 {
          tunnel: w345 -> [w353 w368 w379 w392 w405]
          tunnel: [w355 w369 w381 w394 w407] -> w344
          tunnel: w342 -> [w354 w366 w380 w393 w406]
          frame "Open", "Standard", Default {
            w348 = T3."Standard" ("State")
            n145 = property class="VI"(reference=w354, error in=w353) -> (reference out=w351:refnum<vi>, error out=w352:errorcluster, "FP.State"=w350:T3)
            n146 = Not Equal?(x=w350, y=w348) -> (x != y?=w349:bool)
            n147 = case shown="True" w349 {
              tunnel: [w359 w361] -> w355
              tunnel: w352 -> [w358 w361]
              tunnel: w351 -> [w357 _]
              tunnel: w348 -> [w356 _]
              frame True {
                n148 = invoke class="VI" method="FP.Open"(reference=w357, error in=w358, "Activate"=TRUE, "State"=w356) -> (error out=w359:errorcluster)  [unwired: 1 in, 4 out]
              }
              frame False {
              }
            }
          }
          frame "Close", "Closed" {
            n149 = property class="VI"(reference=w366, error in=w368) -> (reference out=w365:refnum<vi>, error out=w367:errorcluster, "FP.State"=w363:T3)
            n150 = Not Equal?(x=w363, y=T3."Closed" ("Front Panel Window:State")) -> (x != y?=w362:bool)
            n151 = case shown="True" w362 {
              tunnel: [w370 w373] -> w369
              tunnel: w367 -> [w370 w372]
              tunnel: w365 -> [_ w371]
              frame False {
              }
              frame True {
                n152 = invoke class="VI" method="FP.Close"(reference=w371, error in=w372) -> (error out=w373:errorcluster)  [unwired: 1 in, 2 out]
              }
            }
          }
          frame "Hidden", "Hide" {
            w374 = T3."Hidden" ("State")
            n153 = property class="VI"(reference=w380, error in=w379) -> (reference out=w377:refnum<vi>, error out=w378:errorcluster, "FP.State"=w376:T3)
            n154 = Not Equal?(x=w376, y=w374) -> (x != y?=w375:bool)
            n155 = case shown="True" w375 {
              tunnel: [w385 w386] -> w381
              tunnel: w378 -> [w384 w386]
              tunnel: w377 -> [w383 _]
              tunnel: w374 -> [w382 _]
              frame True {
                n156 = invoke class="VI" method="FP.Open"(reference=w383, error in=w384, "State"=w382) -> (error out=w385:errorcluster)  [unwired: 2 in, 4 out]
              }
              frame False {
              }
            }
          }
          frame "Minimize", "Minimized" {
            w387 = T3."Minimized" ("State")
            n157 = property class="VI"(reference=w393, error in=w392) -> (reference out=w390:refnum<vi>, error out=w391:errorcluster, "FP.State"=w389:T3)
            n158 = Not Equal?(x=w389, y=w387) -> (x != y?=w388:bool)
            n159 = case shown="True" w388 {
              tunnel: [w398 w399] -> w394
              tunnel: w391 -> [w397 w399]
              tunnel: w390 -> [w396 _]
              tunnel: w387 -> [w395 _]
              frame True {
                n160 = invoke class="VI" method="FP.Open"(reference=w396, error in=w397, "State"=w395) -> (error out=w398:errorcluster)  [unwired: 2 in, 4 out]
              }
              frame False {
              }
            }
          }
          frame "Maximize", "Maximized" {
            w400 = T3."Maximized" ("State")
            n161 = property class="VI"(reference=w406, error in=w405) -> (reference out=w403:refnum<vi>, error out=w404:errorcluster, "FP.State"=w402:T3)
            n162 = Not Equal?(x=w402, y=w400) -> (x != y?=w401:bool)
            n163 = case shown="True" w401 {
              tunnel: [w411 w412] -> w407
              tunnel: w404 -> [w410 w412]
              tunnel: w403 -> [w409 _]
              tunnel: w400 -> [w408 _]
              frame True {
                n164 = invoke class="VI" method="FP.Open"(reference=w409, error in=w410, "State"=w408) -> (error out=w411:errorcluster)  [unwired: 2 in, 4 out]
              }
              frame False {
              }
            }
          }
        }
        n165 = call <vilib>:"Add State(s) to Queue__JKI_lib_State_Machine.vi"("State(s) in (\"\")"=w347) -> ("States Out"=w346:string)  [unwired: 14 in]
      }
      frame "---------- Macro ----------" {
        # "Do not put any code in this frame.\n(It is a separator no-op. You can make a copy of this frame to create a new Macro frame)"
        n166 = call <vilib>:"Add State(s) to Queue__JKI_lib_State_Machine.vi"("State(s) in (\"\")"=w417) -> ("States Out"=w416:string)  [unwired: 14 in]
      }
      frame "Macro: Initialize" {
        n167 = call <vilib>:"Add State(s) to Queue__JKI_lib_State_Machine.vi"("State(s) in Front (\"\")"="Data: Initialize\nInitialize Core Data\nEvents: Register\nUI: Initialize\n// UI: Front Panel State >> Open\n\n\nAction: Read Config\nAction: Update Indicators\n", "State(s) in (\"\")"=w423) -> ("States Out"=w422:string)  [unwired: 13 in]
      }
      frame "Macro: Update" {
        n168 = call <vilib>:"Add State(s) to Queue__JKI_lib_State_Machine.vi"("State(s) in Front (\"\")"="Action: Update Indicators\nAction: Write Config", "State(s) in (\"\")"=w429) -> ("States Out"=w428:string)  [unwired: 13 in]
      }
      frame "Macro: Exit" {
        # "Exit Macro\n(This is called once, when the VI exits)"
        n169 = Unbundle By Name(w438) -> ("Core.Close Panel on Exit?"=w437:bool)
        n170 = Select(t="UI: Front Panel State >> Close", s=w437, f="") -> (s? t:f=w434:string)
        n171 = call <vilib>:"Add State(s) to Queue__JKI_lib_State_Machine.vi"("State(s) in Front (\"\")"="Action: Write Config", "State(s) in (\"\")"=w434, "State(s) at Back (\"\")"="Data: Cleanup\nEvents: Unregister\nExit") -> ("States Out"=w432:string)  [unwired: 12 in]
        n172 = call <vilib>:"Add State(s) to Queue__JKI_lib_State_Machine.vi"("State(s) in Front (\"\")"=w432, "State(s) in (\"\")"=w441) -> ("States Out"=w440:string)  [unwired: 13 in]
      }
      frame "---------- Action ----------" {
      }
      frame "Action: Read Config" {
        n173 = call "Read ConfigInterface.vi"("GUI in"=w450) -> ()  [unwired: 9 in, 2 out]
        n174 = call <vilib>:"Add State(s) to Queue__JKI_lib_State_Machine.vi"("State(s) in (\"\")"=w446) -> ("States Out"=w447:string)  [unwired: 14 in]
      }
      frame "Action: Write Config" {
      }
      frame "Action: Update Indicators" {
      }
      frame "Action: Update Channels TBL" {
      }
    }
  }
  n175 = call "Read SVW.vi"("GUI in"=w2) -> ("SharedVariableWrapper.lvclass"=w1:refnum<class "SharedVariableWrapper.lvclass">)  [unwired: 10 in]
  n176 = while {
    tunnel: w1 -> [w474]
    shift-right: [w466] -> _
    shift-left: _ -> [w465]
    shift-left: _ -> [w464]
    stop <- "stop" stop-if-true
    n177 = Subtract(x=w465, y=w464) -> ()  [unwired: 1 out]
    n178 = stacked-sequence {
      tunnel: w474 -> [w481 w483 w487 w506 w511]
      tunnel: [w478 _ _ _ _] -> w473
      tunnel: [_ w482 _ _ _] -> w470
      tunnel: [_ _ w486 _ _] -> w469
      tunnel: [_ _ _ w505 _] -> w468
      tunnel: [_ _ _ _ w512] -> w467
      frame #0 {
        n179 = call "Read.vim"("SharedVariableWrapper in"=w481, "name"="DI_ARRAY", "DataType"=bool[] []) -> ("data out"=w477:bool[], "error out"=w478:errorcluster)  [unwired: 6 in, 5 out]
        n180 = Index Array(array=w477) -> ()  [unwired: 12 in, 12 out]
      }
      frame #1 {
        n181 = call "Read.vim"("SharedVariableWrapper in"=w483, "name"="DO_ARRAY", "DataType"=bool[] [] ("appended array")) -> ("error out"=w482:errorcluster)  [unwired: 6 in, 6 out]
      }
      frame #2 {
        n182 = call "Read.vim"("SharedVariableWrapper in"=w487, "name"="AO_ARRAY", "DataType"=dbl[] [] ("appended array")) -> ("error out"=w486:errorcluster)  [unwired: 6 in, 6 out]
      }
      frame #3 {
        n183 = call "Read.vim"("SharedVariableWrapper in"=w506, "name"="NV_1_DATA", "DataType"=T8 {"Engine State"=8, "StateValveModbus"=enum."STOPED", "Alarms"={"OL"=FALSE, "TF"=FALSE, "STL"=FALSE, "OCP"=FALSE, "CPUV"=FALSE, "UVLO"=FALSE, "SPI_ERROR"=FALSE, "Fault"=FALSE, "OL 2"=FALSE, "TF 2"=FALSE, "STL 2"=FALSE, "OCP 2"=FALSE, "CPUV 2"=FALSE, "UVLO 2"=FALSE, "reserved"=TRUE, "InitDone"=TRUE}, "RAW"=124110, "Angele"=0.0, "Step"=0, "Encoder"=0, "Kinematic"={"ACC Steps Per Sec^2"=100, "DEC Steps Per Sec^2"=100, "Min Velosity Step Per Sec"=100, "Max Velosity Step Per Sec"=200, "MicroStep"=16}, "Limits"={"Fault 2 Switch"=FALSE, "Fault 1 Switch"=FALSE, "Center(Home)"=FALSE, "Lower Limit"=FALSE, "Upper Limit"=FALSE}, "EncoderMax"=0, "Counter Max Dont Update"=0, "EncoderMin"=0, "Counter Min Dont Update"=0, "Prepere Counter"=0, "STEP INIT"=0, "offset - Angel"=0.0} ("NVM Data")) -> ("data out"=w509:T8, "error out"=w505:errorcluster)  [unwired: 6 in, 5 out]
        n184 = Unbundle By Name(w509) -> ("Alarms"=w504:T11)
        n185 = Unbundle By Name(w504) -> ("OL"=w503:bool, "TF"=w502:bool, "STL"=w501:bool, "OCP"=w500:bool, "CPUV"=w499:bool, "UVLO"=w498:bool, "SPI_ERROR"=w497:bool, "Fault"=w496:bool, "OL 2"=w495:bool, "TF 2"=w494:bool, "STL 2"=w493:bool, "OCP 2"=w492:bool, "CPUV 2"=w491:bool, "UVLO 2"=w490:bool)  [unwired: 2 out]
        n186 = Compound Arithmetic op=OR(w503, w502, w501, w500, w499, w498, w497, w496, w495, w494, w493, w492, w491, w490) -> ()  [unwired: 1 out]
      }
      frame #4 {
        n187 = call "Read.vim"("SharedVariableWrapper in"=w511, "name"="AI_ARRAY", "DataType"=T14 [] ("AI_Data_Array")) -> ("data out"=w518:T14, "error out"=w512:errorcluster)  [unwired: 6 in, 5 out]
        n188 = Index Array(array=w518, index #1=5 ("index")) -> (element #1=w517:T15, element #2=w515:T15)  [unwired: 1 in]
        n189 = Unbundle By Name(w517) -> ("Stat Data.scl mean 1Hz"=w516:dbl)
        n190 = Unbundle By Name(w515) -> ("Stat Data.scl mean 1Hz"=w514:dbl)
        n191 = local read "Setpoint"() -> (w510:dbl)
        n192 = Bundle("Setpoint"=w510, "scl mean 1Hz"=w516, "scl mean 1Hz"=w514) -> (→"Waveform Chart":T17)  [unwired: 1 in]
      }
    }
    n193 = Merge Errors(w467, w468, w469, w470, w473) -> (w472:errorcluster)
    n194 = Unbundle By Name(w472) -> ("status"=→"Connect":bool)
    n195 = Wait Until Next ms Multiple(millisecond multiple=u32 100) -> (millisecond timer value=w466:u32)
  }
  n196 = flat-sequence {
    tunnel: w7 -> [w523]
    frame #0 {
      n197 = local write "stop"(TRUE ("stop")) -> ()
      "error out" <- w523
    }
  }
